vi "emi_SMLoop Reg QSM.vi"(5 "Loop ID":u16, 9 "error in (no error)":errorcluster) -> (6 "Loop ID Out":u16, 10 "error out":errorcluster)   [LabVIEW 2011]
doc: "Registers a Qued state machine as a SMLoop"
uses:
  Loop control/Private/_emi_Loop control int action.ctl
  Loop control/Private/_emi_GFV Loop Running.vi
  Loop control/Private/_emi_GFV stop a loop so it can reset.vi
  Private/_emi_ SMLoop Restart.vi
  Loop control/Private/_emi_GFV Loop Linking.vi
  Loop control/Private/_emi_GFV Loop Enable.vi
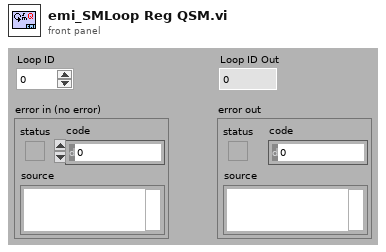
[diagram p1: front panel]
types:
  T1 = typedef "_emi_Loop control int action.ctl" = enum16{"Init index", "Get index", "Set index", "Get Size"}
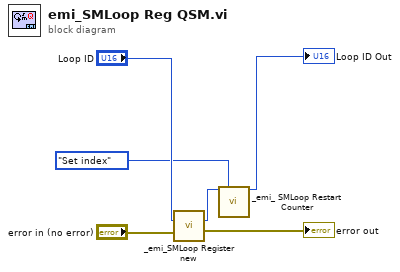
[diagram p0: block diagram]
diagram:
  n1 = call "_emi_SMLoop Register new.vi"("Loop ID"="Loop ID", "error in (no error)"="error in (no error)") -> ("Loop ID Out"=w3:u16, "error out"=→"error out":errorcluster)  [unwired: 12 in]
  n2 = call "_emi_ SMLoop Restart Counter.vi"("Loop Index/Numb"=w3, "Action(Get Index)"=_emi_Loop_control_int_action."Set index") -> ("Index out"=→"Loop ID Out":u16)  [unwired: 11 in, 2 out]
